vi "Define Communication Protocol.vi"(8 "error in (no error)":errorcluster, 11 "Wi-Fi Communication in":refnum<class "Wi-Fi Communication.lvclass">) -> (0 "error out":errorcluster, 3 "Wi-Fi Communication out":refnum<class "Wi-Fi Communication.lvclass">)   [LabVIEW 2020, in "Wi-Fi Communication.lvclass"]
uses:
  Wi-Fi Communication.lvclass
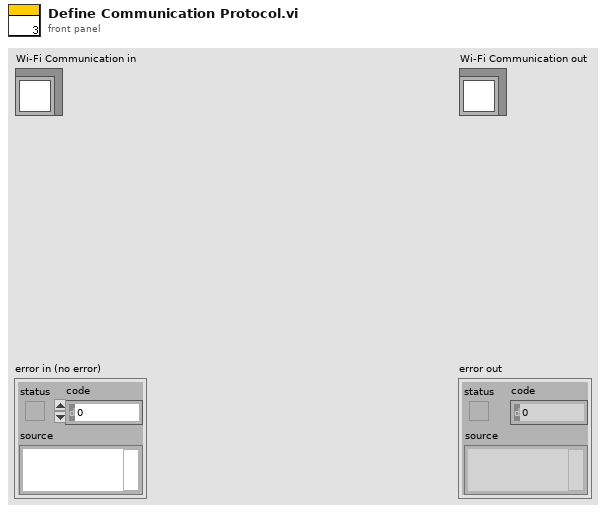
[diagram p1: front panel]
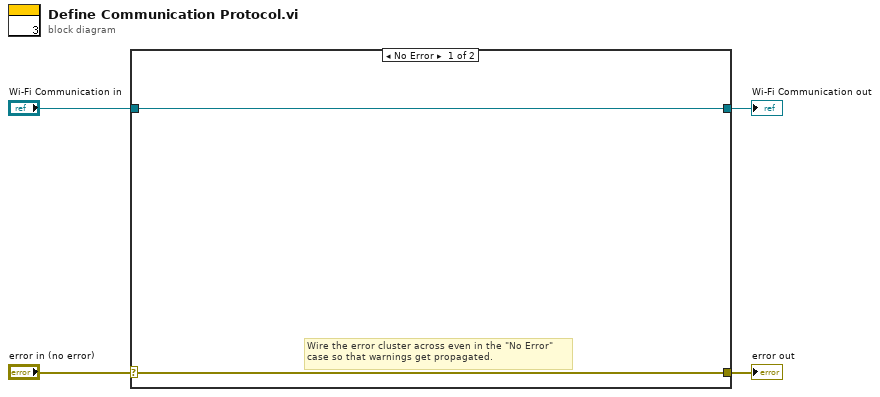
[diagram p0: block diagram]
diagram:
  n1 = case shown="No Error" "error in (no error)" {
    selector: "error in (no error)" -> [w5 w8]
    tunnel: [w5 w8] -> w3
    tunnel: [w6 w7] -> w1
    tunnel: "Wi-Fi Communication in" -> [w6 w7]
    frame No Error {
      # "Wire the error cluster across even in the \"No Error\"\ncase so that warnings get propagated."
    }
    frame Error {
    }
  }
  "error out" <- w3
  "Wi-Fi Communication out" <- w1
